vi "TEMOCR-Parse Response Frame.vi"(9 "pts/pulse":i32, 10 "pulses/frame":i32, 11 "Array in":dbl[](array[numeric])) -> (3 "Array out":dbl[](array[numeric]))   [LabVIEW 2015]
uses:
  <vilib>/Analysis/baseanly.llb/Mean (DBL).vi
  <vilib>/Analysis/NI_AALBase.lvlib
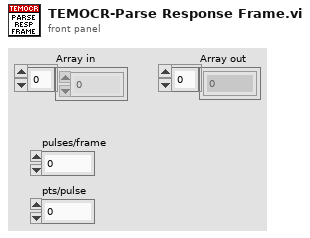
[diagram p1: front panel]
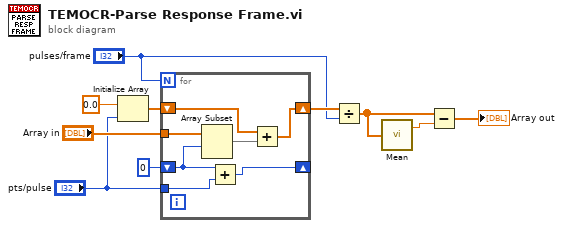
[diagram p0: block diagram]
diagram:
  n1 = Initialize Array(0.0, "pts/pulse") -> (w6:dbl[])
  n2 = for {
    N: "pulses/frame" -> [_]
    tunnel: "Array in" -> [w17]
    shift-right: [w15] -> _
    shift-left: 0 -> [w16]
    tunnel: "pts/pulse" -> [w14]
    shift-right: [w12] -> w5
    shift-left: w6 -> [w11]
    n3 = Array Subset(array=w17, index=w16) -> (w13:dbl[])  [unwired: 1 in]
    n4 = Add(x=w16, y=w14) -> (x+y=w15:i32)
    n5 = Add(x=w11, y=w13) -> (x+y=w12:dbl[])
  }
  n6 = Divide(x=w5, y="pulses/frame") -> (x/y=w2:dbl[])
  n7 = call-poly <vilib>:"Mean.vi"("X"=w2) -> ("mean"=w3:dbl)  [unwired: 1 out]
  n8 = Subtract(x=w2, y=w3) -> (x-y=→"Array out":dbl[])
